vi "3.vi"() -> ()   [LabVIEW 2021]
uses:
  <vilib>/gmath/NI_AAL_MathFunc.lvlib
panel:
  out "Prime Factors":i64[](array[numeric])
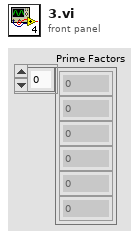
[diagram p1: front panel]
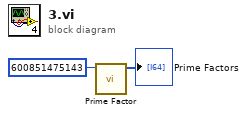
[diagram p0: block diagram]
diagram:
  n1 = call <vilib>:"Prime Factor.vi"("n"=i64 600851475143) -> ("Prime Factors"=→"Prime Factors":i64[])  [unwired: 9 in]
